vi "White Balance.vi"(0 "wRed":u16, 1 "wGreen":u16, 2 "wBlue":u16, 3 "fRelR":sgl, 4 "fRelB":sgl, 5 "info":T1, 7 "error in (no error)":errorcluster) -> (20 "wRed out":u16, 21 "wGreen out":u16, 22 "wBlue out":u16, 23 "fRelR out":sgl, 24 "fRelB out":sgl, 25 "info out":T1, 26 "function return":u32, 27 "error out":errorcluster)   [LabVIEW 2014, in "atmcd32d.lvlib"]
doc: "unsigned int WINAPI WhiteBalance(WORD * wRed, WORD * wGreen, WORD * wBlue, float * fRelR, float * fRelB, WhiteBalanceInfo * info);"
uses:
  atmcd32d.lvlib
  atmcd32d.dll
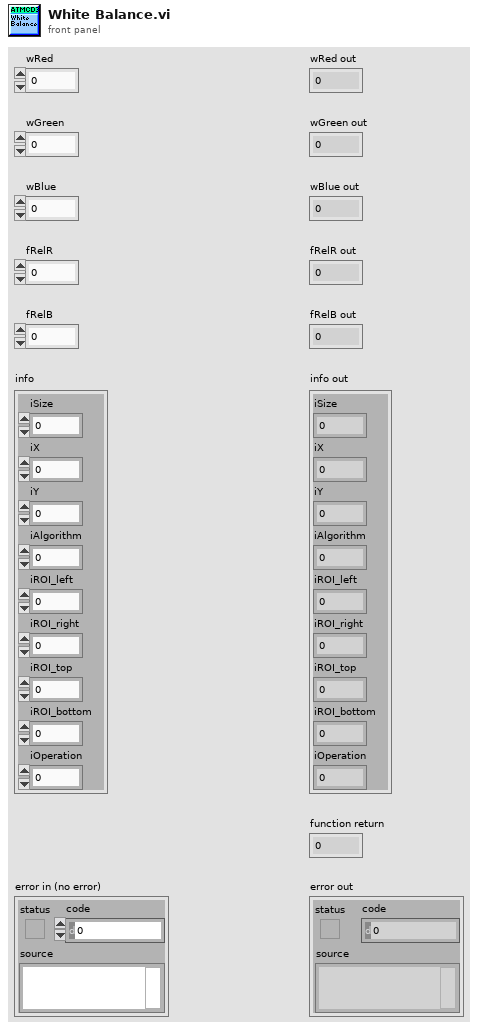
[diagram p1: front panel]
types:
  T1 = cluster{"iSize":i32, "iX":i32, "iY":i32, "iAlgorithm":i32, "iROI_left":i32, "iROI_right":i32, "iROI_top":i32, "iROI_bottom":i32, "iOperation":i32}
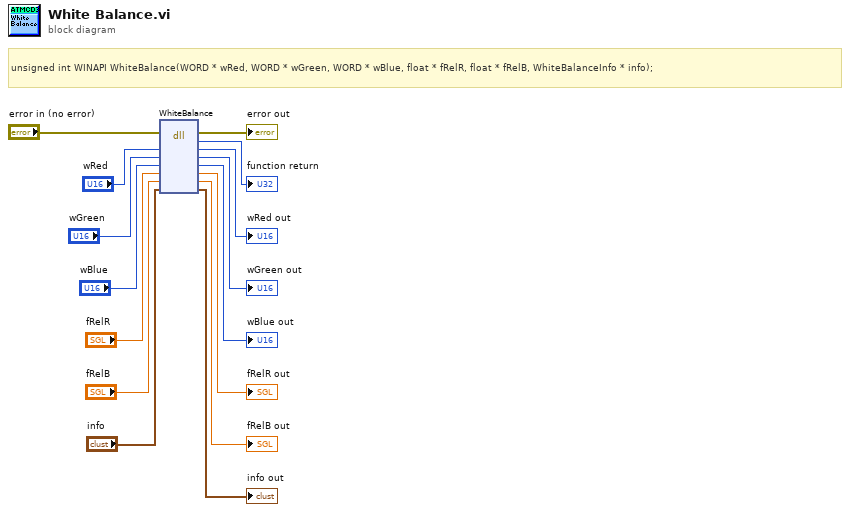
[diagram p0: block diagram]
diagram:
  # "unsigned int WINAPI WhiteBalance(WORD * wRed, WORD * wGreen, WORD * wBlue, float * fRelR, float * fRelB, WhiteBalanceInfo * info);"
  n1 = dll-call lib="C:/Users/Bakir/Documents/Lambda2-Testing/lib/Andorlib/atmcd32d.*" fn="WhiteBalance"(error in="error in (no error)", "wRed"="wRed", "wGreen"="wGreen", "wBlue"="wBlue", "fRelR"="fRelR", "fRelB"="fRelB", "info"="info") -> (error out=→"error out":errorcluster, →"function return":u32, "wRed"=→"wRed out":u16, "wGreen"=→"wGreen out":u16, "wBlue"=→"wBlue out":u16, "fRelR"=→"fRelR out":sgl, "fRelB"=→"fRelB out":sgl, "info"=→"info out":T1)  [unwired: 2 in, 1 out]
